vi "TA_Plot_SelectedKinetics_2.vi"(8 "Selected\nWavelength (nm)":dbl[](array[numeric])=[432.0, 534.0, 643.0], 9 "TA Data":T1={"DeltaA (mOD)"=array424x778[329872 elements], "Wavelength (nm)"=[343.4, 344.2, 344.9, 345.7, 346.5, 347.3, 348.1, 348.9, 349.7, 350.4, 351.2, 352.0, 352.8, 353.6, 354.4, 355.2, 355.9, 356.7, 357.5, 358.3, 359.1, 359.9, 360.7, 361.4, 362.2, 363.0, 363.8, 364.6, 365.4, 366.2, 366.9, 367.7, 368.5, 369.3, 370.1, 370.9, 371.7, 372.5, 373.2, 374.0, 374.8, 375.6, 376.4, 377.2, 378.0, 378.7, 379.5, 380.3, 381.1, 381.9, 382.7, 383.5, 384.2, 385.0, 385.8, 386.6, 387.4, 388.2, 389.0, 389.7, 390.5, 391.3, 392.1, 392.9, 393.7, 394.5, 395.2, 396.0, 396.8, 397.6, 398.4, 399.2, 400.0, 400.7, 401.5, 402.3, 403.1, 403.9, 404.7, 405.5, 406.2, 407.0, 407.8, 408.6, 409.4, 410.2, 411.0, 411.8, 412.5, 413.3, 414.1, 414.9, 415.7, 416.5, 417.3, 418.0, 418.8, 419.6, 420.4, 421.2, 422.0, 422.8, 423.5, 424.3, 425.1, 425.9, 426.7, 427.5, 428.3, 429.0, 429.8, 430.6, 431.4, 432.2, 433.0, 433.8, 434.5, 435.3, 436.1, 436.9, 437.7, 438.5, 439.3, 440.0, 440.8, 441.6, 442.4, 443.2, 444.0, 444.8, 445.5, 446.3, 447.1, 447.9, 448.7, 449.5, 450.3, 451.1, 451.8, 452.6, 453.4, 454.2, 455.0, 455.8, 456.6, 457.3, 458.1, 458.9, 459.7, 460.5, 461.3, 462.1, 462.8, 463.6, 464.4, 465.2, 466.0, 466.8, 467.6, 468.3, 469.1, 469.9, 470.7, 471.5, 472.3, 473.1, 473.8, 474.6, 475.4, 476.2, 477.0, 477.8, 478.6, 479.3, 480.1, 480.9, 481.7, 482.5, 483.3, 484.1, 484.8, 485.6, 486.4, 487.2, 488.0, 488.8, 489.6, 490.4, 491.1, 491.9, 492.7, 493.5, 494.3, 495.1, 495.9, 496.6, 497.4, 498.2, 499.0, 499.8, 500.6, 501.4, 502.1, 502.9, 503.7, 504.5, 505.3, 506.1, 506.9, 507.6, 508.4, 509.2, 510.0, 510.8, 511.6, 512.4, 513.1, 513.9, 514.7, 515.5, 516.3, 517.1, 517.9, 518.6, 519.4, 520.2, 521.0, 521.8, 522.6, 523.4, 524.1, 524.9, 525.7, 526.5, 527.3, 528.1, 528.9, 529.7, 530.4, 531.2, 532.0, 532.8, 533.6, 534.4, 535.2, 535.9, 536.7, 537.5, 538.3, 539.1, 539.9, 540.7, 541.4, 542.2, 543.0, 543.8, 544.6, 545.4, 546.2, 546.9, 547.7, 548.5, 549.3, 550.1, 550.9, 551.7, 552.4, 553.2, 554.0, 554.8, 555.6, 556.4, 557.2, 557.9, 558.7, 559.5, 560.3, 561.1, 561.9, 562.7, 563.4, 564.2, 565.0, 565.8, 566.6, 567.4, 568.2, 569.0, 569.7, 570.5, 571.3, 572.1, 572.9, 573.7, 574.5, 575.2, 576.0, 576.8, 577.6, 578.4, 579.2, 580.0, 580.7, 581.5, 582.3, 583.1, 583.9, 584.7, 585.5, 586.2, 587.0, 587.8, 588.6, 589.4, 590.2, 591.0, 591.7, 592.5, 593.3, 594.1, 594.9, 595.7, 596.5, 597.2, 598.0, 598.8, 599.6, 600.4, 601.2, 602.0, 602.7, 603.5, 604.3, 605.1, 605.9, 606.7, 607.5, 608.3, 609.0, 609.8, 610.6, 611.4, 612.2, 613.0, 613.8, 614.5, 615.3, 616.1, 616.9, 617.7, 618.5, 619.3, 620.0, 620.8, 621.6, 622.4, 623.2, 624.0, 624.8, 625.5, 626.3, 627.1, 627.9, 628.7, 629.5, 630.3, 631.0, 631.8, 632.6, 633.4, 634.2, 635.0, 635.8, 636.5, 637.3, 638.1, 638.9, 639.7, 640.5, 641.3, 642.0, 642.8, 643.6, 644.4, 645.2, 646.0, 646.8, 647.6, 648.3, 649.1, 649.9, 650.7, 651.5, 652.3, 653.1, 653.8, 654.6, 655.4, 656.2, 657.0, 657.8, 658.6, 659.3, 660.1, 660.9, 661.7, 662.5, 663.3, 664.1, 664.8, 665.6, 666.4, 667.2, 668.0, 668.8, 669.6, 670.3, 671.1, 671.9, 672.7, 673.5, 674.3, 675.1, 675.8], "Time (ps)"=array[778 elements], "Size of DeltaA"=[], "Size of Wavelength"=0, "Size of Time"=0}) -> (2 "TA Selected Kinetics":cluster{"Array":dbl[], "Array 2":dbl[]}[](graph), 3 "Selected Kinetics":dbl[][](array[numeric]))   [LabVIEW 2025]
uses:
  TA_DATA.ctl
panel:
  out "Actual Selected Wavelength":dbl[](array[numeric])
  out "DeltaA for Selected Wavelength":dbl[][](array[numeric])
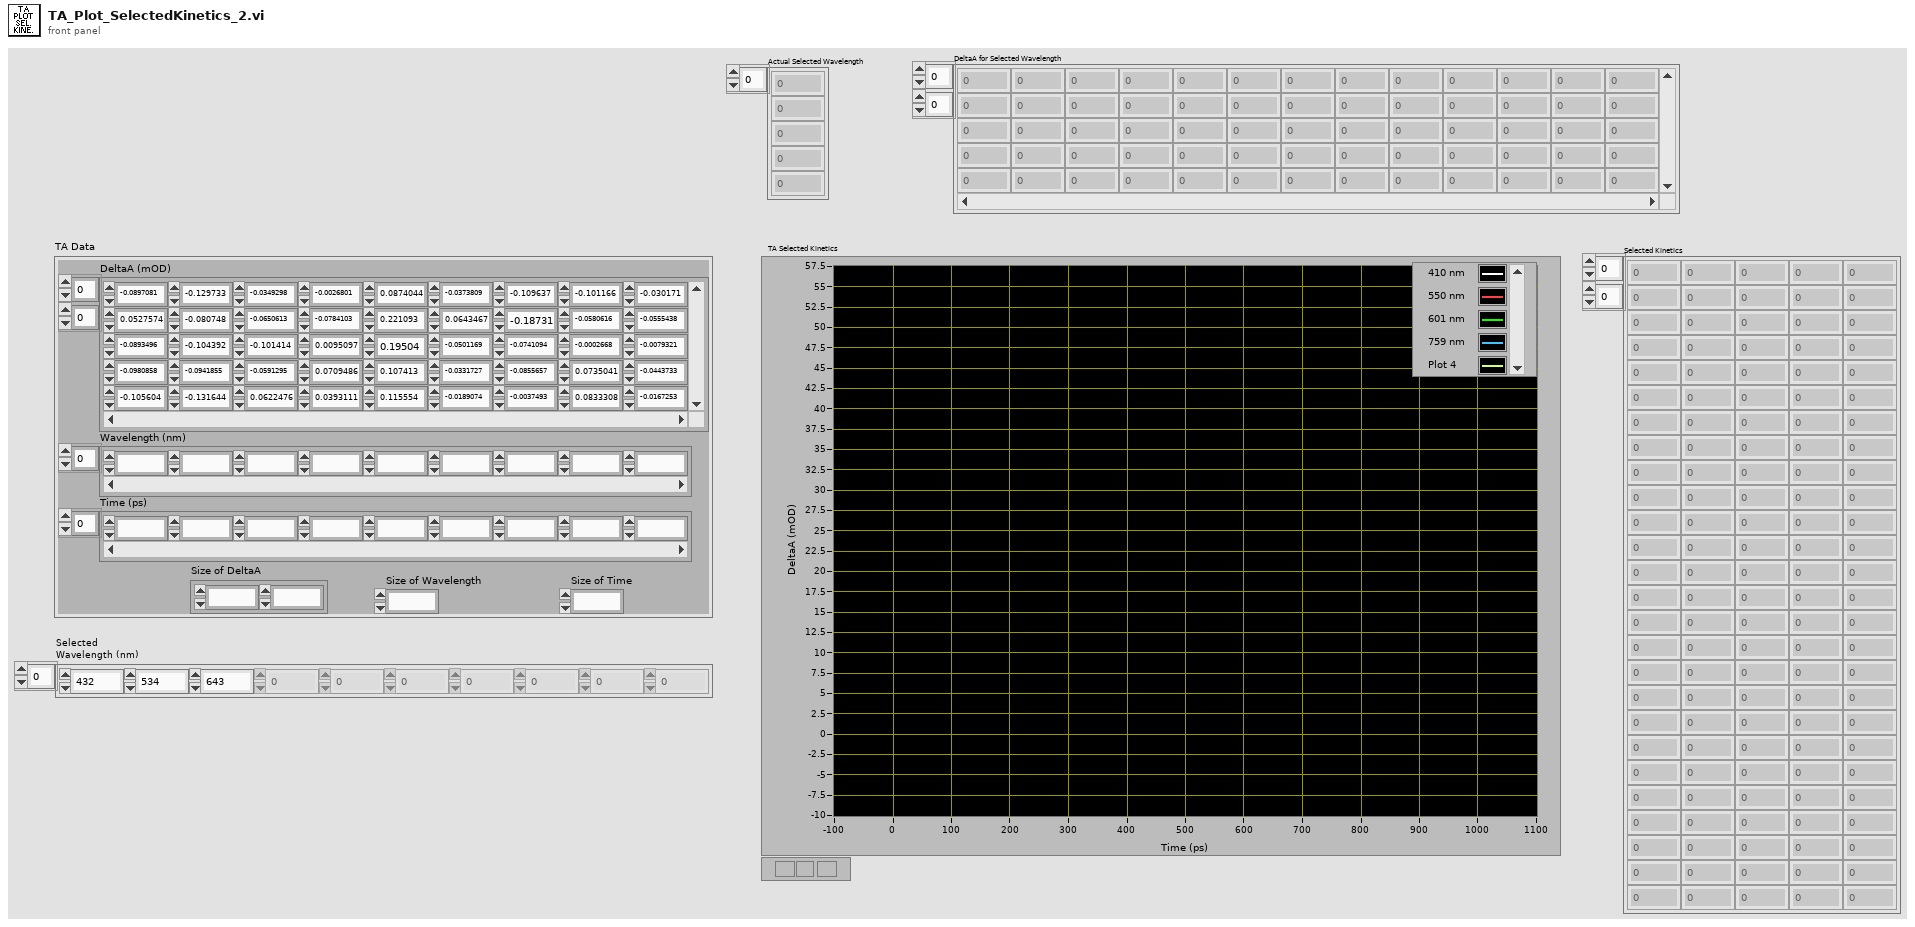
[diagram p1: front panel]
types:
  T1 = typedef "TA_DATA.ctl" = cluster{"DeltaA (mOD)":dbl[][], "Wavelength (nm)":dbl[], "Time (ps)":dbl[], "Size of DeltaA":i32[], "Size of Wavelength":i32, "Size of Time":i32}
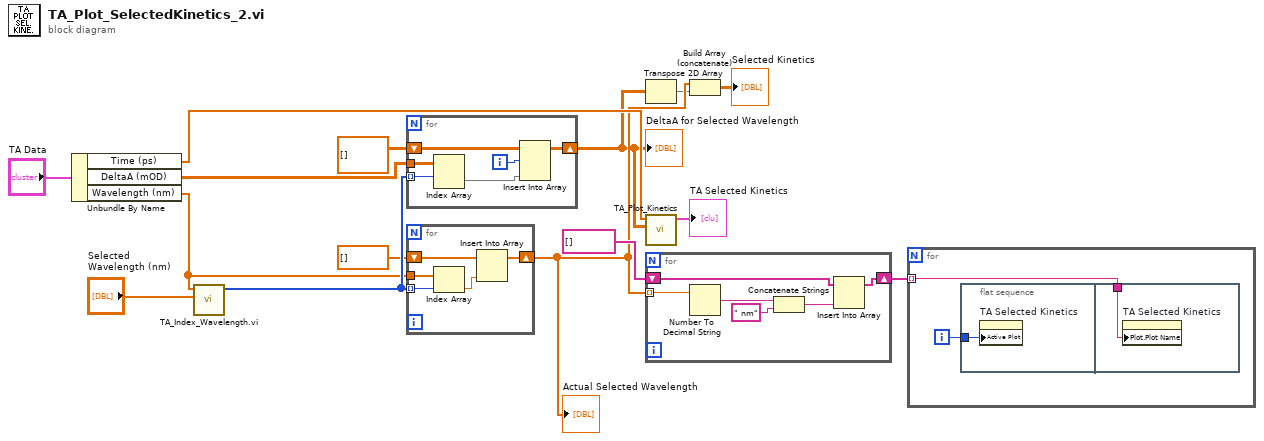
[diagram p0: block diagram]
diagram:
  n1 = Unbundle By Name("TA Data") -> ("Time (ps)"=w12:dbl[], "DeltaA (mOD)"=w3:dbl[][], "Wavelength (nm)"=w1:dbl[])
  n2 = call "TA_Index_Wavelength.vi.vi"("Selected Wavelength"="Selected\nWavelength (nm)", "Wavelength (nm)"=w1) -> ("Index of Selected Wavelength"=w13:i32[])  [unwired: 9 in]
  n3 = for {
    shift-right: [w19] -> w5
    shift-left: dbl[][] [] ("Array") -> [w21]
    tunnel: w13 -> [w18] mode=indexing
    tunnel: w3 -> [w16]
    i -> [w17]
    n4 = Index Array(array=w16, index (row)=w18) -> (element=w20:dbl[])  [unwired: 1 in]
    n5 = Insert Into Array(array=w21, index (row)=w17, new element=w20) -> (w19:dbl[][])  [unwired: 1 in]
  }
  "DeltaA for Selected Wavelength" <- w5
  n6 = for {
    shift-right: [w25] -> w6
    shift-left: dbl[] [] ("Array") -> [w24]
    tunnel: w13 -> [w26] mode=indexing
    tunnel: w1 -> [w23]
    n7 = Index Array(array=w23, index=w26) -> (element=w22:dbl)
    n8 = Insert Into Array(array=w24, new element=w22) -> (w25:dbl[])  [unwired: 1 in]
  }
  "Actual Selected Wavelength" <- w6
  n9 = Transpose 2D Array(2D array=w5) -> (transposed array=w4:dbl[][])
  n10 = call "TA_Plot_Kinetics.vi"("DeltaA (mOD)"=w5, "Time (ps)"=w12) -> ("TA Kinetics"=→"TA Selected Kinetics":cluster{"Array":dbl[], "Array 2":dbl[]}[])  [unwired: 9 in]
  n11 = for {
    tunnel: w6 -> [w32] mode=indexing
    shift-right: [w27] -> w8
    shift-left: string[] [] ("Array") -> [w28]
    n12 = Number To Decimal String(number=w32) -> (decimal integer string=w30:string)  [unwired: 1 in]
    n13 = Concatenate Strings(w30, " nm" ("string")) -> (w29:string)
    n14 = Insert Into Array(array=w28, new element=w29) -> (w27:string[])  [unwired: 1 in]
  }
  n15 = Build Array (concatenate)(w6, w4) -> (→"Selected Kinetics":dbl[][])
  n16 = for {
    tunnel: w8 -> [w34] mode=indexing
    i -> [w33]
    n17 = flat-sequence {
      tunnel: w33 -> [w35]
      tunnel: w34 -> [w36]
      frame #0 {
        n18 = property on="TA Selected Kinetics" class="XYGraph (strict)"("Active Plot"=w35) -> ()  [unwired: 2 in, 2 out]
      }
      frame #1 {
        n19 = property on="TA Selected Kinetics" class="XYGraph (strict)"("Plot.Plot Name"=w36) -> ()  [unwired: 2 in, 2 out]
      }
    }
  }
